vi "elaborateData.vi"(0 "reference in":refnum<class "Subject Controller.lvclass">, 2 "data":string[][][](array[string]), 5 "error in (no error)":errorcluster) -> (14 "reference out":refnum<class "Subject Controller.lvclass">, 19 "error out":errorcluster)   [LabVIEW 2015, in "Subject Controller.lvclass"]
uses:
  Subject Controller.lvclass
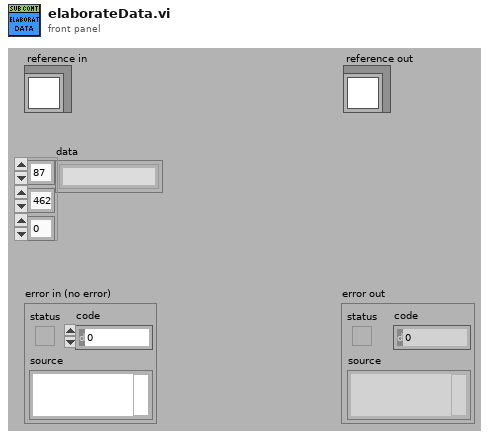
[diagram p1: front panel]
types:
  T1 = typedef "Subject Controller.lvclass/ObjectAttributesRef.ctl" = refnum<data-value>
  T2 = typedef "Subject Controller.lvclass/ObjectAttributes.ctl" = cluster{"MyAttribute":dbl, "subject_controller_ref":refnum<class "Subject Controller.lvclass">, "file_controller_ref":refnum<class "File Controller.lvclass">, "subject_refs":refnum<class "subject.lvclass">[], "subjectIndex":i32, "file_type":T3}
  T3 = typedef "excelFile.lvclass/fileType.ctl" = enum16{"database", "CosmedTest"}
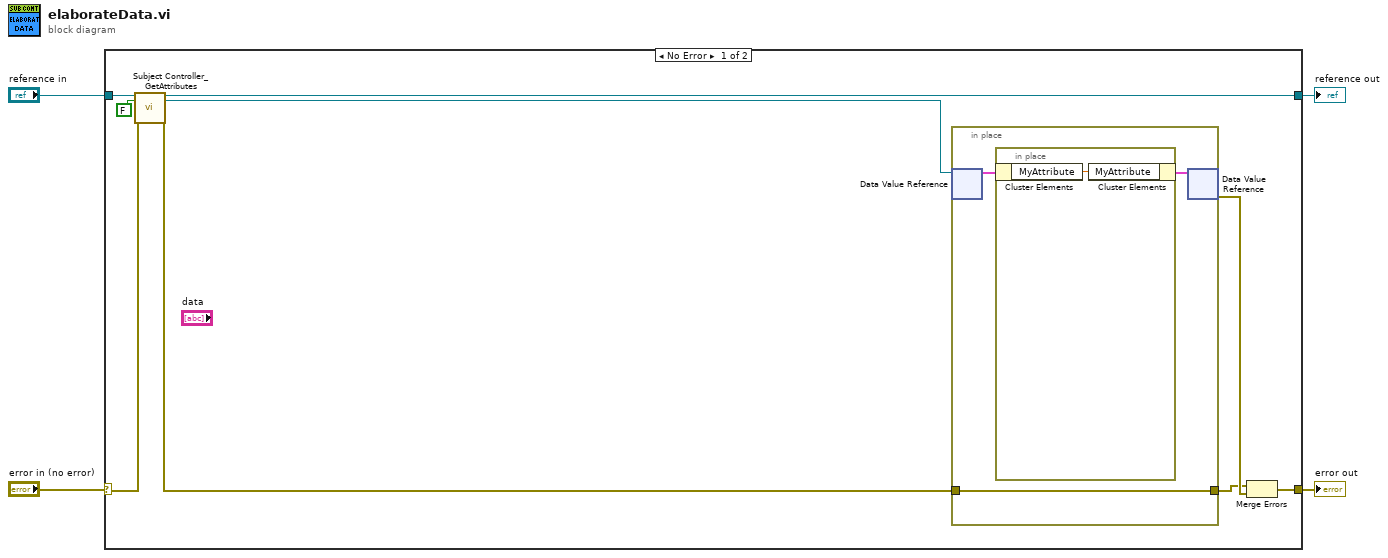
[diagram p0: block diagram]
diagram:
  n1 = case shown="No Error" "error in (no error)" {
    selector: "error in (no error)" -> [w8 w19]
    tunnel: [w13 w19] -> w3
    tunnel: [w6 w18] -> w1
    tunnel: "reference in" -> [w10 w18]
    frame No Error {
      n2 = call "Subject Controller_GetAttributes.vi"("reference in"=w10, "return data? (T)"=FALSE, "error in (no error)"=w8) -> ("reference out"=w6:refnum<class "Subject Controller.lvclass">, "attributes ref"=w5:T1, "error out"=w7:errorcluster)  [unwired: 13 in, 1 out]
      n3 = in-place {
        in-place-border: w7 -> [w14]
        in-place-border: [w14] -> w11
        n4 = in-place-dvr #1(w5) -> (w15:T2)  [unwired: 1 out]
        n5 = in-place {
          n6 = in-place-cluster #2(w15) -> ("MyAttribute"=w17:dbl)
          n7 = in-place-cluster #2("MyAttribute"=w17) -> (w16:T2)
        }
        n8 = in-place-dvr #1(w16) -> (w12:errorcluster)  [unwired: 1 out]
      }
      n9 = Merge Errors(w11, w12) -> (w13:errorcluster)
    }
    frame Error {
    }
  }
  "error out" <- w3
  "reference out" <- w1
